vi "5-digits_display_driver.vi"(10 "precision":u8=2, 11 "number":dbl=156.72 format="%#.10f") -> (2 "OF":bool, 3 "Display":T1)   [LabVIEW 2015]
doc: "This module is a 5-digit 7-segment display driver, plus an additional digit on the left to display the letter E as an error indication (at the user's discretion), and to display the minus sign.\n<b>number</b> is any real number between -99999 and 99999, it is a floating point number.\n<b>precision</b> is the number of decimal places to display.\n<b>Display</b> is the display itself.\n<b>OF</b> is the overflow indicator in case number is outside the range indicated above."
uses:
  controls/green 5-digit display.ctl
  controls/green 7-seg display.ctl
  controls/green 7-seg display special.ctl
panel:
  # "5-digits display driver with overflow"
  # "OverFlow"
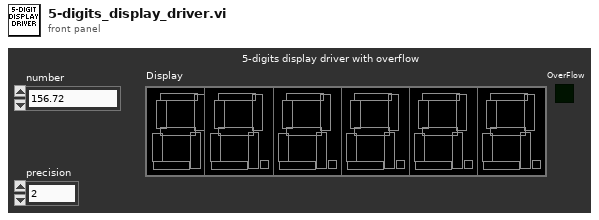
[diagram p1: front panel]
types:
  T1 = typedef "green 5-digit display.ctl" = cluster{"digit_1":T2, "digit_2":T2, "digit_3":T2, "digit_4":T2, "digit_5":T2, "special":T3}
  T2 = typedef "green 7-seg display.ctl" = cluster{"a-seg":bool, "b-seg":bool, "c-seg":bool, "d-seg":bool, "e-seg":bool, "f-seg":bool, "g-seg":bool, "dp-seg":bool}
  T3 = typedef "green 7-seg display special.ctl" = cluster{"a-seg":bool, "b-seg":bool, "c-seg":bool, "d-seg":bool, "e-seg":bool, "f-seg":bool, "g-seg":bool}
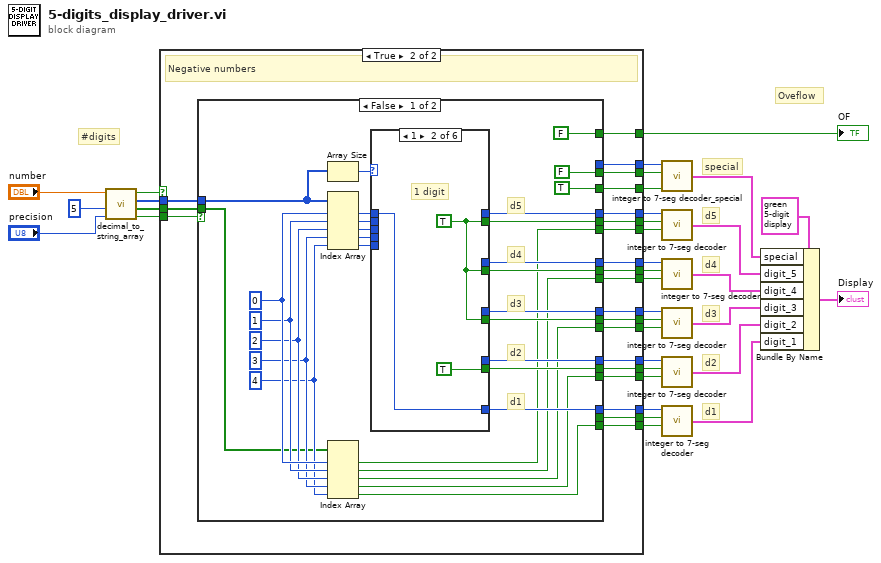
[diagram p0: block diagram]
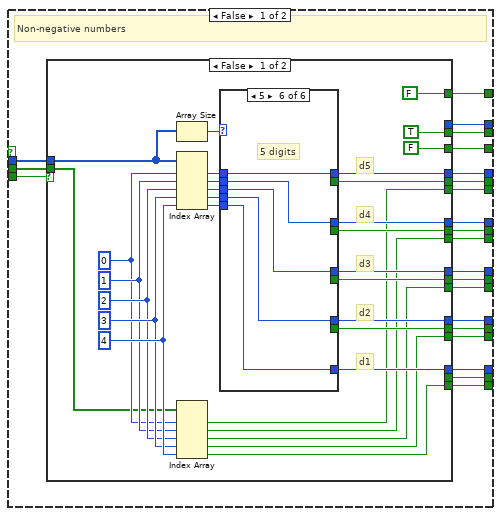
[diagram p2: hidden frame]
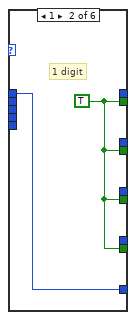
[diagram p4: hidden frame]
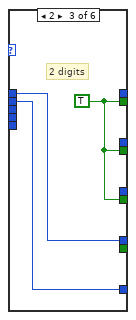
[diagram p5: hidden frame]
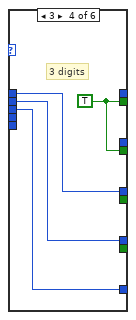
[diagram p6: hidden frame]
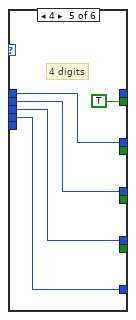
[diagram p7: hidden frame]
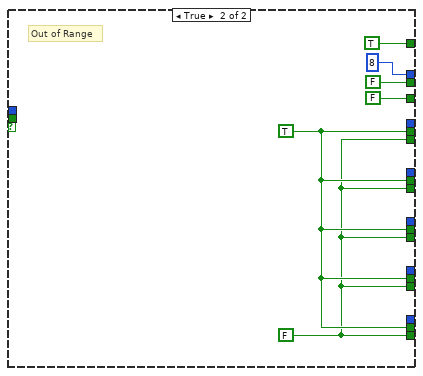
[diagram p8: hidden frame]
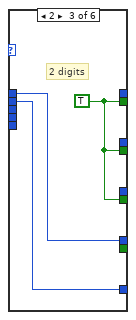
[diagram p10: hidden frame]
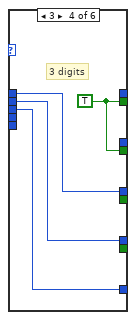
[diagram p11: hidden frame]
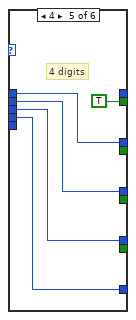
[diagram p12: hidden frame]
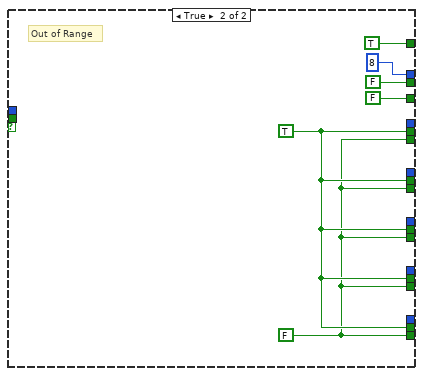
[diagram p14: hidden frame]
diagram:
  # "#digits"
  # "Oveflow"
  # "d5"
  # "d4"
  # "d3"
  # "d2"
  # "d1"
  # "special"
  n1 = call "decimal_to_string_array.vi"("precision"="precision", "No. of display digits"=5, "number in"="number") -> ("out of range?"=w12:bool, "dot position"=w11:bool[], "number array"=w10:u16[], "negative?"=w9:bool)  [unwired: 5 in]
  n2 = case shown="True" w9 {
    tunnel: w12 -> [w56 w117]
    tunnel: [w55 w132] -> w34
    tunnel: [w54 w121] -> w33
    tunnel: [w53 w122] -> w32
    tunnel: [w52 w125] -> w31
    tunnel: [w51 w128] -> w30
    tunnel: [w50 w131] -> w29
    tunnel: [w49 w119] -> w28
    tunnel: [w48 w118] -> w27
    tunnel: [w47 w123] -> w26
    tunnel: [w46 w126] -> w25
    tunnel: [w45 w129] -> w24
    tunnel: [w44 w116] -> w23
    tunnel: [w43 w124] -> w22
    tunnel: [w42 w127] -> w21
    tunnel: [w41 w130] -> w20
    tunnel: [w40 w120] -> w19
    tunnel: w10 -> [w39 w133]
    tunnel: w11 -> [w38 w115]
    tunnel: [w37 w114] -> w7
    tunnel: [w36 w113] -> w6
    tunnel: [w35 w112] -> w4
    frame False {
      # "Non-negative numbers"
      n3 = case shown="False" w56 {
        tunnel: [FALSE TRUE] -> w55
        tunnel: [w79 _] -> w54
        tunnel: [w78 _] -> w53
        tunnel: [w77 _] -> w52
        tunnel: [w76 _] -> w51
        tunnel: [w75 _] -> w50
        tunnel: [w57 w109] -> w49
        tunnel: [w58 w109] -> w48
        tunnel: [w59 w109] -> w47
        tunnel: [w60 w109] -> w46
        tunnel: [w61 w109] -> w45
        tunnel: [w71 w110] -> w44
        tunnel: [w72 w110] -> w43
        tunnel: [w73 w110] -> w42
        tunnel: [w74 w110] -> w41
        tunnel: [_ w110] -> w40
        tunnel: w39 -> [w68 _]
        tunnel: w38 -> [w62 _]
        tunnel: [TRUE FALSE] -> w37
        tunnel: [FALSE FALSE] -> w36
        tunnel: [_ u16 8 ("Integer number")] -> w35
        frame False {
          w67 = 4 ("index")
          w66 = 3 ("index")
          w65 = 2 ("index")
          w64 = 1 ("index")
          w63 = 0 ("index")
          # "d5"
          # "d4"
          # "d3"
          # "d2"
          # "d1"
          n4 = Array Size(array=w68) -> (size(s)=w85:i32)
          n5 = Index Array(array=w68, index #1=w63, index #2=w64, index #3=w65, index #4=w66, index #5=w67) -> (element #1=w80:u16, element #2=w81:u16, element #3=w82:u16, element #4=w83:u16, element #5=w84:u16)
          n6 = Index Array(array=w62, index #1=w63, index #2=w64, index #3=w65, index #4=w66, index #5=w67) -> (element #1=w61:bool, element #2=w60:bool, element #3=w59:bool, element #4=w58:bool, element #5=w57:bool)
          n7 = case shown="5" w85 {
            tunnel: w84 -> [_ _ _ _ _ w101]
            tunnel: w83 -> [_ _ _ _ w97 w102]
            tunnel: w82 -> [_ _ _ w93 w98 w103]
            tunnel: w81 -> [_ _ w90 w94 w96 w104]
            tunnel: w80 -> [_ w88 w91 w95 w99 w105]
            tunnel: [_ w88 w90 w93 w97 w101] -> w79
            tunnel: [_ _ w91 w94 w98 w102] -> w78
            tunnel: [_ _ _ w95 w96 w103] -> w77
            tunnel: [_ _ _ _ w99 w104] -> w76
            tunnel: [_ _ _ _ _ w105] -> w75
            tunnel: [_ w87 w89 w92 TRUE _] -> w74
            tunnel: [_ w87 w89 w92 _ _] -> w73
            tunnel: [_ w87 w89 _ _ _] -> w72
            tunnel: [_ w87 _ _ _ _] -> w71
            frame 0, Default {
            }
            frame 1 {
              w87 = TRUE
              # "1 digit"
            }
            frame 2 {
              w89 = TRUE
              # "2 digits"
            }
            frame 3 {
              w92 = TRUE
              # "3 digits"
            }
            frame 4 {
              # "4 digits"
            }
            frame 5 {
              # "5 digits"
            }
          }
        }
        frame True {
          w109 = FALSE
          w110 = TRUE
          # "Out of Range"
        }
      }
    }
    frame True {
      # "Negative numbers"
      n8 = case shown="False" w117 {
        tunnel: [FALSE TRUE] -> w132
        tunnel: [w156 _] -> w121
        tunnel: [w155 _] -> w122
        tunnel: [w154 _] -> w125
        tunnel: [w153 _] -> w128
        tunnel: [w152 _] -> w131
        tunnel: [w134 w187] -> w119
        tunnel: [w135 w187] -> w118
        tunnel: [w136 w187] -> w123
        tunnel: [w137 w187] -> w126
        tunnel: [w138 w187] -> w129
        tunnel: [w148 w188] -> w116
        tunnel: [w149 w188] -> w124
        tunnel: [w150 w188] -> w127
        tunnel: [w151 w188] -> w130
        tunnel: [_ w188] -> w120
        tunnel: w133 -> [w145 _]
        tunnel: w115 -> [w139 _]
        tunnel: [FALSE FALSE] -> w114
        tunnel: [TRUE FALSE] -> w113
        tunnel: [_ u16 8 ("Integer number")] -> w112
        frame False {
          w140 = 4 ("index")
          w141 = 3 ("index")
          w142 = 2 ("index")
          w143 = 1 ("index")
          w144 = 0 ("index")
          # "d5"
          # "d4"
          # "d3"
          # "d2"
          # "d1"
          n9 = Array Size(array=w145) -> (size(s)=w162:i32)
          n10 = Index Array(array=w145, index #1=w144, index #2=w143, index #3=w142, index #4=w141, index #5=w140) -> (element #1=w157:u16, element #2=w158:u16, element #3=w159:u16, element #4=w160:u16, element #5=w161:u16)
          n11 = Index Array(array=w139, index #1=w144, index #2=w143, index #3=w142, index #4=w141, index #5=w140) -> (element #1=w138:bool, element #2=w137:bool, element #3=w136:bool, element #4=w135:bool, element #5=w134:bool)
          n12 = case shown="1" w162 {
            tunnel: w161 -> [_ _ _ _ _ w179]
            tunnel: w160 -> [_ _ _ _ w176 w180]
            tunnel: w159 -> [_ _ _ w171 w177 w181]
            tunnel: w158 -> [_ _ w168 w172 w175 w182]
            tunnel: w157 -> [_ w166 w169 w173 w178 w183]
            tunnel: [_ w166 w168 w171 w176 w179] -> w156
            tunnel: [_ _ w169 w172 w177 w180] -> w155
            tunnel: [_ _ _ w173 w175 w181] -> w154
            tunnel: [_ _ _ _ w178 w182] -> w153
            tunnel: [_ _ _ _ _ w183] -> w152
            tunnel: [_ w165 w167 w170 TRUE _] -> w151
            tunnel: [_ w165 w167 w170 _ _] -> w150
            tunnel: [_ w165 w167 _ _ _] -> w149
            tunnel: [_ TRUE _ _ _ _] -> w148
            frame 0, Default {
            }
            frame 1 {
              w165 = TRUE
              # "1 digit"
            }
            frame 2 {
              w167 = TRUE
              # "2 digits"
            }
            frame 3 {
              w170 = TRUE
              # "3 digits"
            }
            frame 4 {
              # "4 digits"
            }
            frame 5 {
              # "5 digits"
            }
          }
        }
        frame True {
          w187 = FALSE
          w188 = TRUE
          # "Out of Range"
        }
      }
    }
  }
  "OF" <- w34
  n13 = call "integer to 7-seg decoder_special.vi"("Integer number"=w4, "Display On/Off"=w7, "Is negative? (F)"=w6) -> ("7-seg digit for negative"=w5:T3)  [unwired: 5 in]
  n14 = call "integer to 7-seg decoder.vi"("Integer number"=w29, "Display On/Off"=w20, "dp"=w24) -> ("7-seg digit"=w18:T2)  [unwired: 5 in]
  n15 = call "integer to 7-seg decoder.vi"("Integer number"=w30, "Display On/Off"=w21, "dp"=w25) -> ("7-seg digit"=w17:T2)  [unwired: 5 in]
  n16 = call "integer to 7-seg decoder.vi"("Integer number"=w31, "Display On/Off"=w22, "dp"=w26) -> ("7-seg digit"=w16:T2)  [unwired: 5 in]
  n17 = call "integer to 7-seg decoder.vi"("Integer number"=w32, "Display On/Off"=w23, "dp"=w27) -> ("7-seg digit"=w15:T2)  [unwired: 5 in]
  n18 = call "integer to 7-seg decoder.vi"("Integer number"=w33, "Display On/Off"=w19, "dp"=w28) -> ("7-seg digit"=w14:T2)  [unwired: 5 in]
  n19 = Bundle By Name(cluster=T1 {"digit_1"={"a-seg"=TRUE, "b-seg"=TRUE, "c-seg"=FALSE, "d-seg"=TRUE, "e-seg"=TRUE, "f-seg"=FALSE, "g-seg"=TRUE, "dp-seg"=FALSE}, "digit_2"={"a-seg"=TRUE, "b-seg"=TRUE, "c-seg"=TRUE, "d-seg"=FALSE, "e-seg"=FALSE, "f-seg"=FALSE, "g-seg"=FALSE, "dp-seg"=FALSE}, "digit_3"={"a-seg"=TRUE, "b-seg"=FALSE, "c-seg"=TRUE, "d-seg"=TRUE, "e-seg"=TRUE, "f-seg"=TRUE, "g-seg"=TRUE, "dp-seg"=TRUE}, "digit_4"={"a-seg"=TRUE, "b-seg"=FALSE, "c-seg"=TRUE, "d-seg"=TRUE, "e-seg"=FALSE, "f-seg"=TRUE, "g-seg"=TRUE, "dp-seg"=FALSE}, "digit_5"={"a-seg"=FALSE, "b-seg"=TRUE, "c-seg"=TRUE, "d-seg"=FALSE, "e-seg"=FALSE, "f-seg"=FALSE, "g-seg"=FALSE, "dp-seg"=FALSE}, "special"={"a-seg"=FALSE, "b-seg"=FALSE, "c-seg"=FALSE, "d-seg"=FALSE, "e-seg"=FALSE, "f-seg"=FALSE, "g-seg"=FALSE}} ("Display"), "special"=w5, "digit_5"=w18, "digit_4"=w17, "digit_3"=w16, "digit_2"=w15, "digit_1"=w14) -> (→"Display":T1)
